vi "Read Test Method Count.vi"(11 "Test Suite Result In":T1) -> (1 "Test Method count string":string, 2 "Test Method count":i32, 3 "Test Suite Result Out":T1)   [LabVIEW 2020, in "Test Suite Result.lvlib"]
uses:
  Test Suite Result.lvlib
  Test Suite Result type.ctl
  Assertion Result/Public/TypeDefs/Status.ctl
  Case Result/Test Case Result type.ctl
  Method Result/Method Result type.ctl
  Assertion Result/Assertion Result type.ctl
  Assertion Result/Public/TypeDefs/Assertion Type.ctl
  Case Result/Test Case Result.lvlib
  Assertion Result/Assertion Result.lvlib
  Method Result/Method Result.lvlib
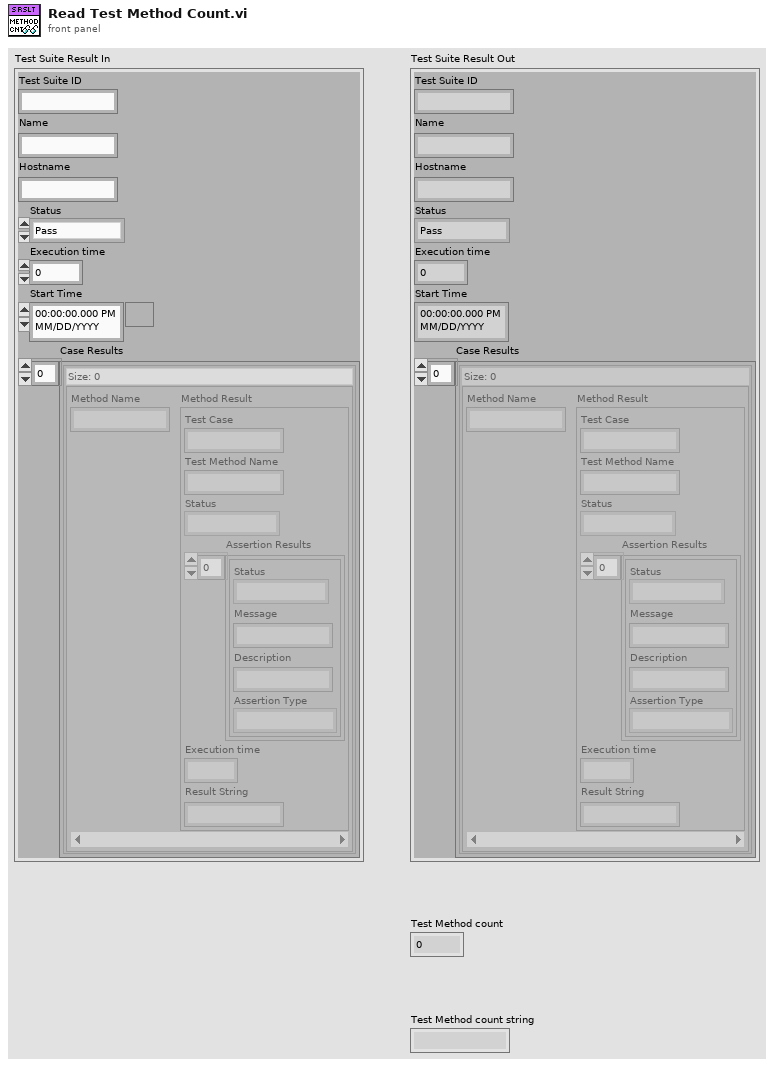
[diagram p1: front panel]
types:
  T1 = typedef "Test Suite Result.lvlib/Test Suite Result type.ctl" = cluster{"Test Suite ID":string, "Name":string, "Hostname":string, "Status":T2, "Execution time":dbl, "Start Time":timestamp, "Case Results":T3[]}
  T2 = typedef "Assertion Result.lvlib/Status.ctl" = enum16{"Pass", "Fail", "Error", "Skipped", "Setup Error", "Broken", "Teardown Error"}
  T3 = typedef "Test Case Result.lvlib/Test Case Result type.ctl" = map{string, T4}
  T4 = typedef "Method Result.lvlib/Method Result type.ctl" = cluster{"Test Case":string, "Test Method Name":string, "Status":T2, "Assertion Results":T5[], "Execution time":dbl, "Result String":string}
  T5 = typedef "Assertion Result.lvlib/Assertion Result type.ctl" = cluster{"Status":T2, "Message":string, "Description":string, "Assertion Type":T6}
  T6 = typedef "Assertion Result.lvlib/Assertion Type.ctl" = enum16{"None", "Pass", "Fail", "Skip", "Pass if Equal", "Fail if Equal", "Pass if Error", "Fail if Error", "Pass if", "Fail if"}
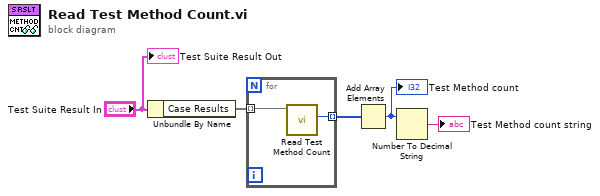
[diagram p0: block diagram]
diagram:
  n1 = Unbundle By Name("Test Suite Result In") -> ("Case Results"=w3:T3[])
  n2 = for {
    tunnel: w3 -> [w7] mode=indexing
    tunnel: [w6] -> w2 mode=indexing
    n3 = call "Read Test Method Count.vi"("Test Case Result In"=w7) -> ("Numeric"=w6:i32)  [unwired: 9 in, 1 out]
  }
  n4 = Add Array Elements(numeric array=w2) -> (sum=w1:i32)
  "Test Method count" <- w1
  n5 = Number To Decimal String(number=w1) -> (decimal integer string=→"Test Method count string":string)  [unwired: 1 in]
  "Test Suite Result Out" <- "Test Suite Result In"
